vi "test Loopback_Acyclic_SelectiveTrigger.vi"(8 "error in":errorcluster, 11 "TestCase in":refnum<class "Single Core Acyclic Loopback.lvclass">) -> (0 "error out":errorcluster, 3 "TestCase out":refnum<class "Single Core Acyclic Loopback.lvclass">)   [LabVIEW 2020, in "Single Core Acyclic Loopback.lvclass"]
uses:
  Single Core Acyclic Loopback.lvclass
  C:/Git/niveristand-custom-device-testing-tools/VeriStandTestCase/VeriStandTestCase.lvclass
  <vilib>/numeric/sub_Random U32.vi
  <vilib>/NI VeriStand/Execution/Workspace/NI VeriStand - Set Multiple Channel Values.vi
  <vilib>/numeric/Random Number (Range) I64.vi
  <vilib>/addons/_JKI Toolkits/VI Tester/TestCase.llb/TestCase.lvclass
  <vilib>/NI VeriStand/Execution/Workspace/NI_VS Workspace ExecutionAPI.lvlib
  C:/Program Files (x86)/National Instruments/LabVIEW 2020/vi.lib/addons/_JKI Toolkits/VI Tester/TestCase.llb/TestCase.lvclass
  C:/Git/niveristand-ballard-arinc429-custom-device/Source/Custom Device Support/Tests/System/Single Core (P2--P3) Acyclic Loopback/Single Core Acyclic Loopback.lvclass
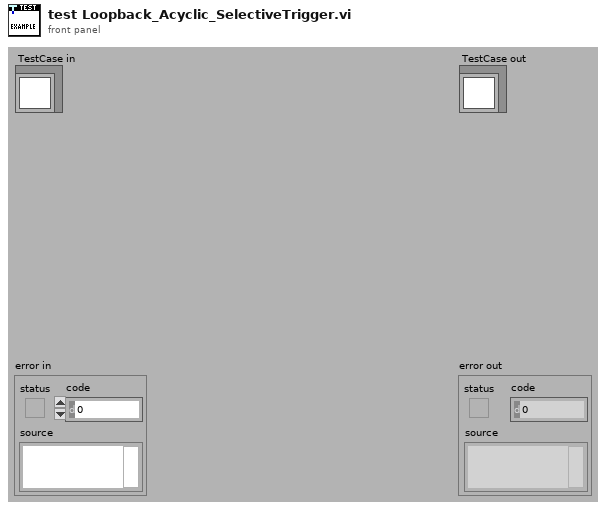
[diagram p1: front panel]
types:
  T1 = typedef "NI_VS Workspace ExecutionAPI.lvlib/WorkspaceAPI.ctl" = refnum<k24>
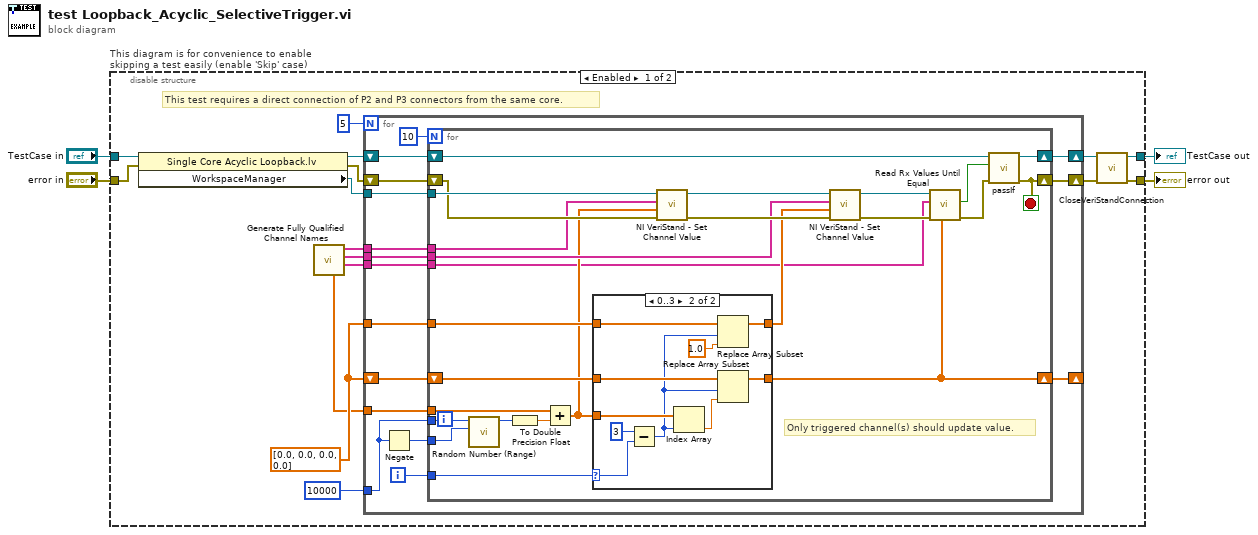
[diagram p0: block diagram]
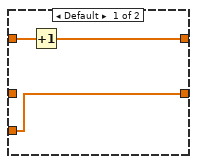
[diagram p2: hidden frame]
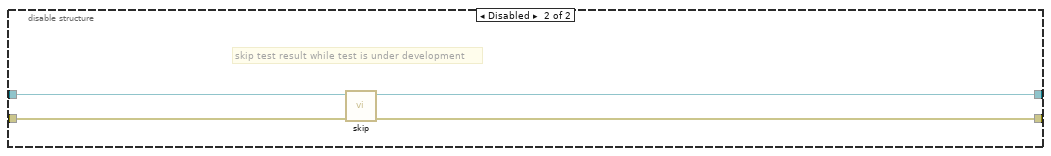
[diagram p3: hidden frame]
diagram:
  n1 = disable-structure "This diagram is for convenience to enable skipping a test easily (enable 'Skip' case)" shown="Enabled" {
    disable-tunnel: "TestCase in" -> [w20 w78]
    disable-tunnel: [w18 w76] -> w1
    disable-tunnel: [w17 w77] -> w3
    disable-tunnel: "error in" -> [w19 w75]
    frame Enabled {
      w9 = dbl[] [0.0, 0.0, 0.0, 0.0] ("Values")
      # "This test requires a direct connection of P2 and P3 connectors from the same core."
      n2 = property class="Single Core Acyclic Loopback.lv"(reference=w20, error in=w19) -> (reference out=w13:refnum<class "Single Core Acyclic Loopback.lvclass">, error out=w14:errorcluster, "WorkspaceManager"=w15:T1)
      n3 = call "Generate Fully Qualified Channel Names.vi"() -> ("Rx channels"=w6:string[], "trigger channels"=w5:string[], "Tx channels"=w8:string[], "channel index"=w7:dbl[])  [unwired: 8 in]
      n4 = for {
        N: 5 -> [_]
        tunnel: w7 -> [w36]
        tunnel: i64 10000 ("upper bound (100)") -> [w35]
        tunnel: w8 -> [w34]
        tunnel: w15 -> [w33]
        tunnel: w6 -> [w31]
        shift-right: [w28] -> w11
        shift-left: w14 -> [w32]
        shift-right: [w29] -> w12
        shift-left: w13 -> [w30]
        tunnel: w5 -> [w26]
        shift-right: [w23] -> _
        shift-left: w9 -> [w25]
        tunnel: w9 -> [w24]
        i -> [w27]
        n5 = Negate(x=w35) -> (-x=w22:i64)
        n6 = for {
          N: 10 -> [_]
          tunnel: w36 -> [w60]
          tunnel: w35 -> [w59]
          tunnel: w22 -> [w58]
          tunnel: w34 -> [w49]
          tunnel: w33 -> [w51]
          tunnel: w31 -> [w37]
          shift-right: [w57] -> w29
          shift-left: w30 -> [w48]
          shift-right: [w56] -> w28
          shift-left: w32 -> [w50]
          tunnel: w27 -> [w46]
          tunnel: w26 -> [w47]
          shift-right: [w38] -> w23
          shift-left: w25 -> [w40]
          tunnel: w24 -> [w41]
          stop <- w56 stop-if-true
          # "Only triggered channel(s) should update value."
          n7 = call-poly <vilib>:"Random Number (Range).vi"("lower bound (-100)"=w58, "upper bound (100)"=w59) -> ("number"=w61:i64)  [unwired: 9 in]
          n8 = To Double Precision Float(number=w61) -> (double precision float=w44:dbl)
          n9 = Add(x=w60, y=w44) -> (x+y=w39:dbl[])
          n10 = case shown="0..3" w46 {
            selector: w46 -> [_ w74]
            tunnel: [w63 w71] -> w45
            tunnel: w41 -> [w64 w70]
            tunnel: w40 -> [_ w69]
            tunnel: w39 -> [w62 w68]
            tunnel: [w62 w66] -> w38
            frame Default {
              n11 = Increment(x=w64) -> (x+1=w63:dbl[])
            }
            frame 0..3 {
              n12 = Subtract(x=3, y=w74) -> (x-y=w65:i32)
              n13 = Index Array(array=w68, index=w65) -> (element=w67:dbl)
              n14 = Replace Array Subset(array=w70, new element=1.0 ("new element/subarray"), index=w65) -> (w71:dbl[])
              n15 = Replace Array Subset(array=w69, new element=w67, index=w65) -> (w66:dbl[])
            }
          }
          n16 = call-poly <vilib>:"NI VeriStand - Set Channel Value.vi"("error in (no error)"=w50, "Values"=w39, "Channels"=w49, "WorkspaceManager in"=w51) -> ("error out"=w52:errorcluster, "WorkspaceManager out"=w55:T1)  [unwired: 6 in]
          n17 = call-poly <vilib>:"NI VeriStand - Set Channel Value.vi"("error in (no error)"=w52, "Values"=w45, "Channels"=w47, "WorkspaceManager in"=w55) -> ("error out"=w53:errorcluster, "WorkspaceManager out"=w54:T1)  [unwired: 6 in]
          n18 = call "Read Rx Values Until Equal.vi"("expected values"=w38, "error in"=w53, "Rx aliases"=w37, "workspace manager in"=w54) -> ("error out"=w42:errorcluster, "values equal expected"=w43:bool)  [unwired: 5 in, 1 out]
          n19 = call-dynamic "passIf.vi"("error in (no error)"=w42, "pass"=w43, "TestCase in"=w48) -> ("error out"=w56:errorcluster, "TestCase out"=w57:refnum<class "Single Core Acyclic Loopback.lvclass">)  [unwired: 7 in]
        }
      }
      n20 = call-dynamic "CloseVeriStandConnection.vi"("error in (no error)"=w11, "VeriStand Test Case in"=w12) -> ("error out"=w17:errorcluster, "VeriStand Test Case out"=w18:refnum<class "Single Core Acyclic Loopback.lvclass">)  [unwired: 8 in]
    }
    frame Disabled {
      # "skip test result while test is under development"
      n21 = call <vilib>:"skip.vi"("error in (no error)"=w75, "TestCase in"=w78) -> ("error out"=w77:errorcluster, "TestCase out"=w76:refnum<class "Single Core Acyclic Loopback.lvclass">)  [unwired: 8 in]
    }
  }
  "error out" <- w3
  "TestCase out" <- w1
